vi "Setting Up.vi"(4 "Async Elements":refnum<class "Async Elements.lvclass">, 6 "VI Ref":refnum<vi>, 7 "Actor in":refnum<class "Actor.lvclass">, 9 "Transport":refnum<class "Transport.lvclass">) -> (0 "Error out":errorcluster, 5 "Actor out":refnum<class "Actor.lvclass">)   [LabVIEW 2020, in "jettl.lvlib"]
uses:
  jettl.lvlib
  Actor/Actor.lvclass
  Transport/Transport.lvclass
  Async Elements/Async Elements.lvclass
  Attributes/Attributes.lvclass
  Teardown Location.ctl
  Async Elements.ctl
  Base Async Elements/Base Async Elements.lvlib
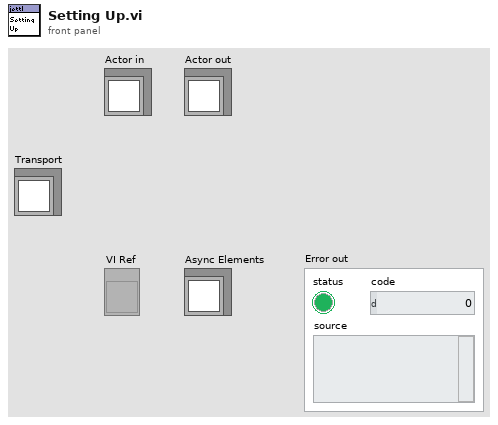
[diagram p1: front panel]
types:
  T1 = typedef "jettl.lvlib/Async Elements.ctl" = cluster{"Attributes":refnum<class "Attributes.lvclass">, "Error":errorcluster}
  T2 = typedef "jettl.lvlib/Teardown Location.ctl" = enum16{"Setting Up", "Tearing Down"}
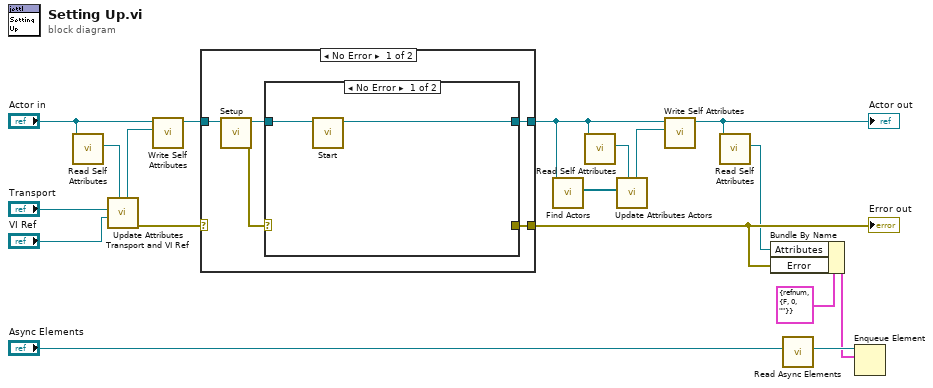
[diagram p0: block diagram]
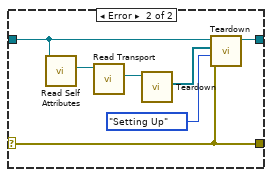
[diagram p2: hidden frame]
diagram:
  n1 = call-dynamic "Read Self Attributes.vi"("Actor in"="Actor in") -> ("Self Attributes"=w4:refnum<class "Attributes.lvclass">)  [unwired: 10 in]
  n2 = call "Update Attributes Transport and VI Ref.vi"("Attributes in"=w4, "VI Ref"="VI Ref", "Transport"="Transport") -> ("Error out"=w2:errorcluster, "Attributes out"=w5:refnum<class "Attributes.lvclass">)  [unwired: 7 in]
  n3 = call-dynamic "Write Self Attributes.vi"("Self Attributes"=w5, "Actor in"="Actor in") -> ("Actor out"=w1:refnum<class "Actor.lvclass">)  [unwired: 9 in]
  n4 = case shown="No Error" w2 {
    selector: w2 -> [_ w33]
    tunnel: [w23 w33] -> w18
    tunnel: [w22 w34] -> w15
    tunnel: w1 -> [w19 w34]
    frame No Error {
      n5 = call-dynamic "Setup.vi"("Actor in"=w19) -> ("Error out"=w20:errorcluster, "Actor out"=w21:refnum<class "Actor.lvclass">)  [unwired: 9 in]
      n6 = case shown="No Error" w20 {
        selector: w20 -> [_ w31]
        tunnel: w21 -> [w25 w28]
        tunnel: [_ w31] -> w23
        tunnel: [w24 w32] -> w22
        frame No Error {
          n7 = call-dynamic "Start.vi"("Actor in"=w25) -> ("Actor out"=w24:refnum<class "Actor.lvclass">)  [unwired: 10 in]
        }
        frame Error {
          n8 = call-dynamic "Read Self Attributes.vi"("Actor in"=w28) -> ("Self Attributes"=w27:refnum<class "Attributes.lvclass">)  [unwired: 10 in]
          n9 = call-dynamic "Read Transport.vi"("Attributes in"=w27) -> ("Transport"=w26:refnum<class "Transport.lvclass">)  [unwired: 10 in]
          n10 = call-dynamic "Teardown.vi"("Transport in"=w26) -> ("Unheard Msgs"=w29:refnum<class "Msg.lvclass">[])  [unwired: 10 in]
          n11 = call-dynamic "Teardown.vi"("Error in"=w31, "Teardown Location"=Teardown_Location."Setting Up", "Unheard Msgs"=w29, "Actor in"=w28) -> ("Actor out"=w32:refnum<class "Actor.lvclass">)  [unwired: 7 in]
        }
      }
    }
    frame Error {
    }
  }
  "Error out" <- w18
  n12 = call-dynamic "Find Actors.vi"("Actor in"=w15) -> ("Actors"=w14:refnum<class "Actor.lvclass">[])  [unwired: 10 in]
  n13 = call-dynamic "Read Self Attributes.vi"("Actor in"=w15) -> ("Self Attributes"=w7:refnum<class "Attributes.lvclass">)  [unwired: 10 in]
  n14 = call "Update Attributes Actors.vi"("Attributes in"=w7, "Actors"=w14) -> ("Attributes out"=w6:refnum<class "Attributes.lvclass">)  [unwired: 9 in]
  n15 = call-dynamic "Write Self Attributes.vi"("Self Attributes"=w6, "Actor in"=w15) -> ("Actor out"=w3:refnum<class "Actor.lvclass">)  [unwired: 9 in]
  "Actor out" <- w3
  n16 = call-dynamic "Read Self Attributes.vi"("Actor in"=w3) -> ("Self Attributes"=w17:refnum<class "Attributes.lvclass">)  [unwired: 10 in]
  n17 = Bundle By Name(cluster=T1 {"Attributes"=refnum, "Error"={"status"=FALSE, "code"=0, "source"=""}} ("element"), "Attributes"=w17, "Error"=w18) -> (w11:T1)
  n18 = call "Read Async Elements.vi"("Async Elements"="Async Elements") -> ("Async Elements"=w12:refnum<queue>)  [unwired: 10 in]
  n19 = Enqueue Element(queue=w12, element=w11) -> ()  [unwired: 2 in, 3 out]
